vi "LIDAR File Saver.vi"   [LabVIEW 2015]
uses:
  LIDAR Globals.vi
types:
  T1 = enum16{"open", "replace", "create", "open or create", "replace or create", "replace or create with confirmation"}
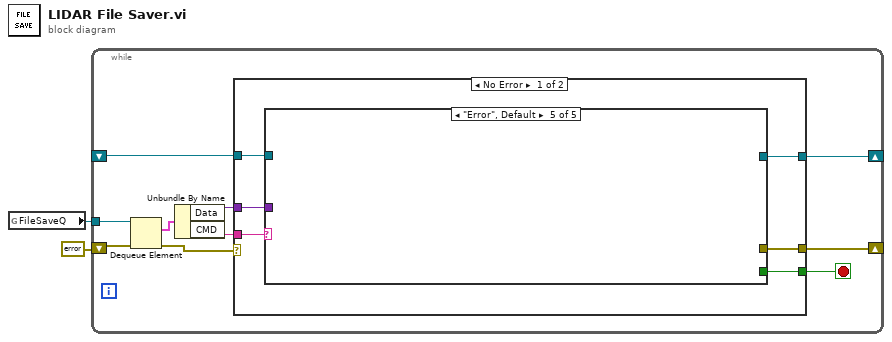
[diagram p0: block diagram]
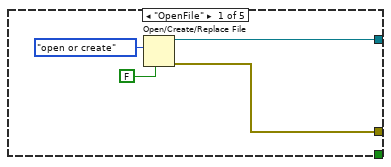
[diagram p2: hidden frame]
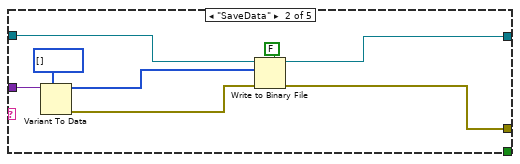
[diagram p3: hidden frame]
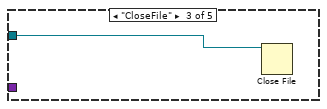
[diagram p4: hidden frame]
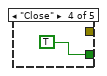
[diagram p5: hidden frame]
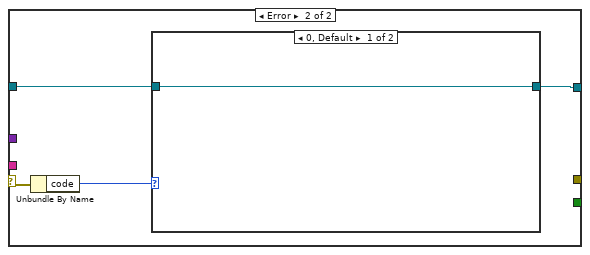
[diagram p6: hidden frame]
diagram:
  n1 = global read "LIDAR Globals.vi" "FileSaveQ"() -> (w1:refnum<queue>)
  n2 = while {
    tunnel: w1 -> [w12]
    shift-right: [w8] -> _
    shift-left: _ -> [w7]
    shift-right: [w5] -> _
    shift-left: errorcluster {"status"=FALSE, "code"=0, "source"=""} ("error out") -> [w4]
    stop <- w9 stop-if-true
    n3 = Dequeue Element(queue=w12, error in (no error)=w4) -> (element=w11:cluster{"CMD":string, "Data":variant}, error out=w3:errorcluster)  [unwired: 1 in, 2 out]
    n4 = Unbundle By Name(w11) -> ("Data"=w6:variant, "CMD"=w10:string)
    n5 = case shown="No Error" w3 {
      selector: w3 -> [_ w36]
      tunnel: w10 -> [w18 _]
      tunnel: [w17 _] -> w9
      tunnel: [w16 w33] -> w8
      tunnel: w7 -> [w15 w34]
      tunnel: w6 -> [w14 _]
      tunnel: [w13 _] -> w5
      frame No Error {
        n6 = case shown="\"Error\", Default" w18 {
          tunnel: [_ _ _ TRUE _] -> w17
          tunnel: [w20 w28 _ _ _] -> w16
          tunnel: w15 -> [_ w29 w31 _ _]
          tunnel: w14 -> [_ w27 _ _ _]
          tunnel: [w19 w24 _ _ _] -> w13
          frame "OpenFile" {
            n7 = Open/Create/Replace File(operation (0:open)=T1."open or create", disable buffering (F)=FALSE) -> (refnum out=w20:refnum<file>, error out=w19:errorcluster)  [unwired: 4 in, 1 out]
          }
          frame "SaveData" {
            n8 = Variant To Data(type=u64[] [] ("Data"), Variant=w27) -> (data=w25:u64[], error out=w23:errorcluster)  [unwired: 1 in]
            n9 = Write to Binary File(file (use dialog)=w29, data=w25, error in=w23, 5:FALSE ("prepend array or string size? (T)")) -> (refnum out=w28:refnum<file>, error out=w24:errorcluster)  [unwired: 2 in, 1 out]
          }
          frame "CloseFile" {
            n10 = Close File(refnum=w31) -> ()  [unwired: 1 in, 2 out]
          }
          frame "Close" {
          }
          frame "Error", Default {
          }
        }
      }
      frame Error {
        n11 = Unbundle By Name(w36) -> ("code"=w35:i32)
        n12 = case shown="0, Default" w35 {
          tunnel: w34 -> [w37 w38]
          tunnel: [w37 w38] -> w33
          frame 0, Default {
          }
          frame 1 {
          }
        }
      }
    }
  }
